vi "MainTester.vi"() -> ()   [LabVIEW 2015]
uses:
  <vilib>/Rock Robotics/WPI/SerialPort/WPI_SerialPortRef.ctl
  <vilib>/Rock Robotics/WPI/SerialPort/WPI_SerialPort.ctl
  Old code/packet types.ctl
panel:
  in  "B 2":dbl(slide) scale=0.0..255.0
  in  "G 2":dbl(slide) scale=0.0..255.0
  in  "R 2":dbl(slide) scale=0.0..255.0
  in  "B":dbl(slide) scale=0.0..255.0
  in  "G":dbl(slide) scale=0.0..255.0
  in  "R":dbl(slide) scale=0.0..255.0
  out "SerialPortRef 6":T1
  out "error out 8":errorcluster
  out "SerialPortRef":T1
  out "error out 7":errorcluster
  in  "Close File 2":bool
  in  "Close File":bool
  in  "Display string":string
  out "error out 6":errorcluster
  out "SerialPortRef 5":T1
  out "ADC voltages":dbl[](array[numeric])
  out "error out 4":errorcluster
  out "SerialPortRef 3":T1
  out "error out 3":errorcluster
  out "SerialPortRef 2":T1
  out "error out 2":errorcluster
  out "All Digital Input Vals":bool[](array[boolean])
  out "error out":errorcluster
  in  "stop":bool
  in  "error in (no error)":errorcluster
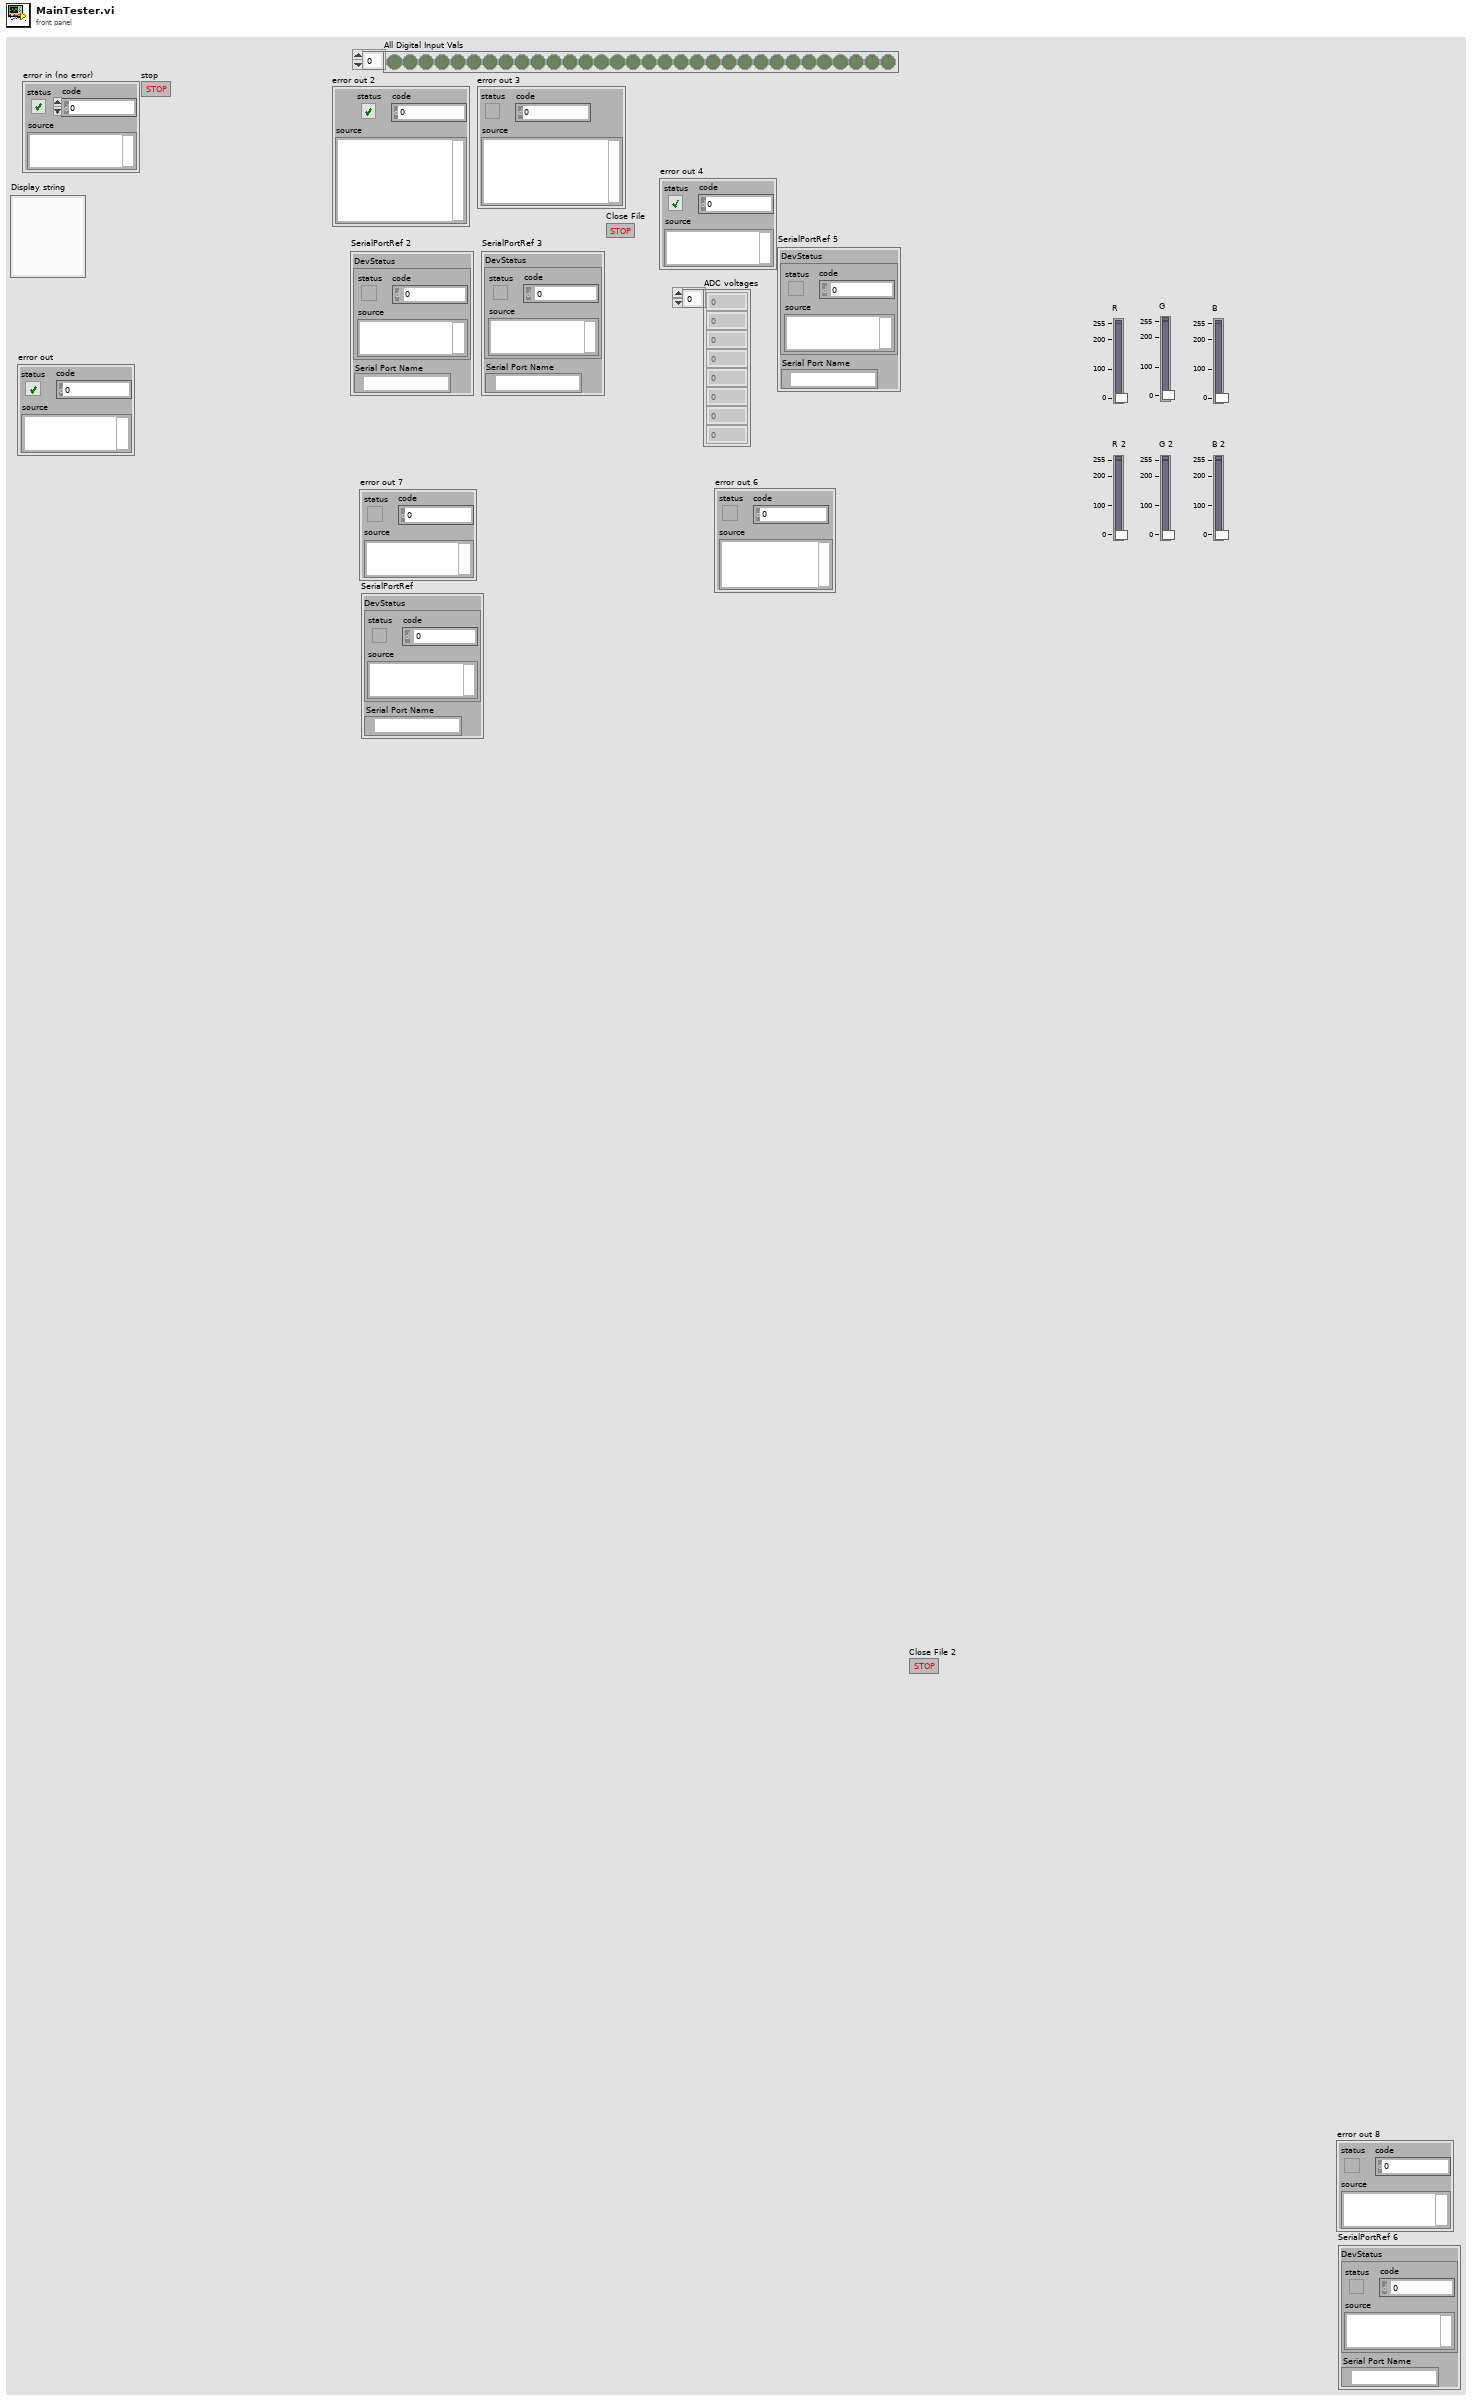
[diagram p1: front panel]
types:
  T1 = typedef "WPI_SerialPortRef.ctl" = cluster{"DevStatus":errorcluster, "Serial Port Name":refnum<visa-resource-name>}
  T2 = typedef "WPI_SerialPort.ctl" = enum16{"Onboard RS-232", "MXP TTL"}
  T3 = typedef "packet types.ctl" = enum16{"Log line", "Open File", "Close File", "Send Header", "Set Time", "Send to LCD"}
  T4 = enum16{"Set Custom RGB", "Set Mode", "Set intensity"}
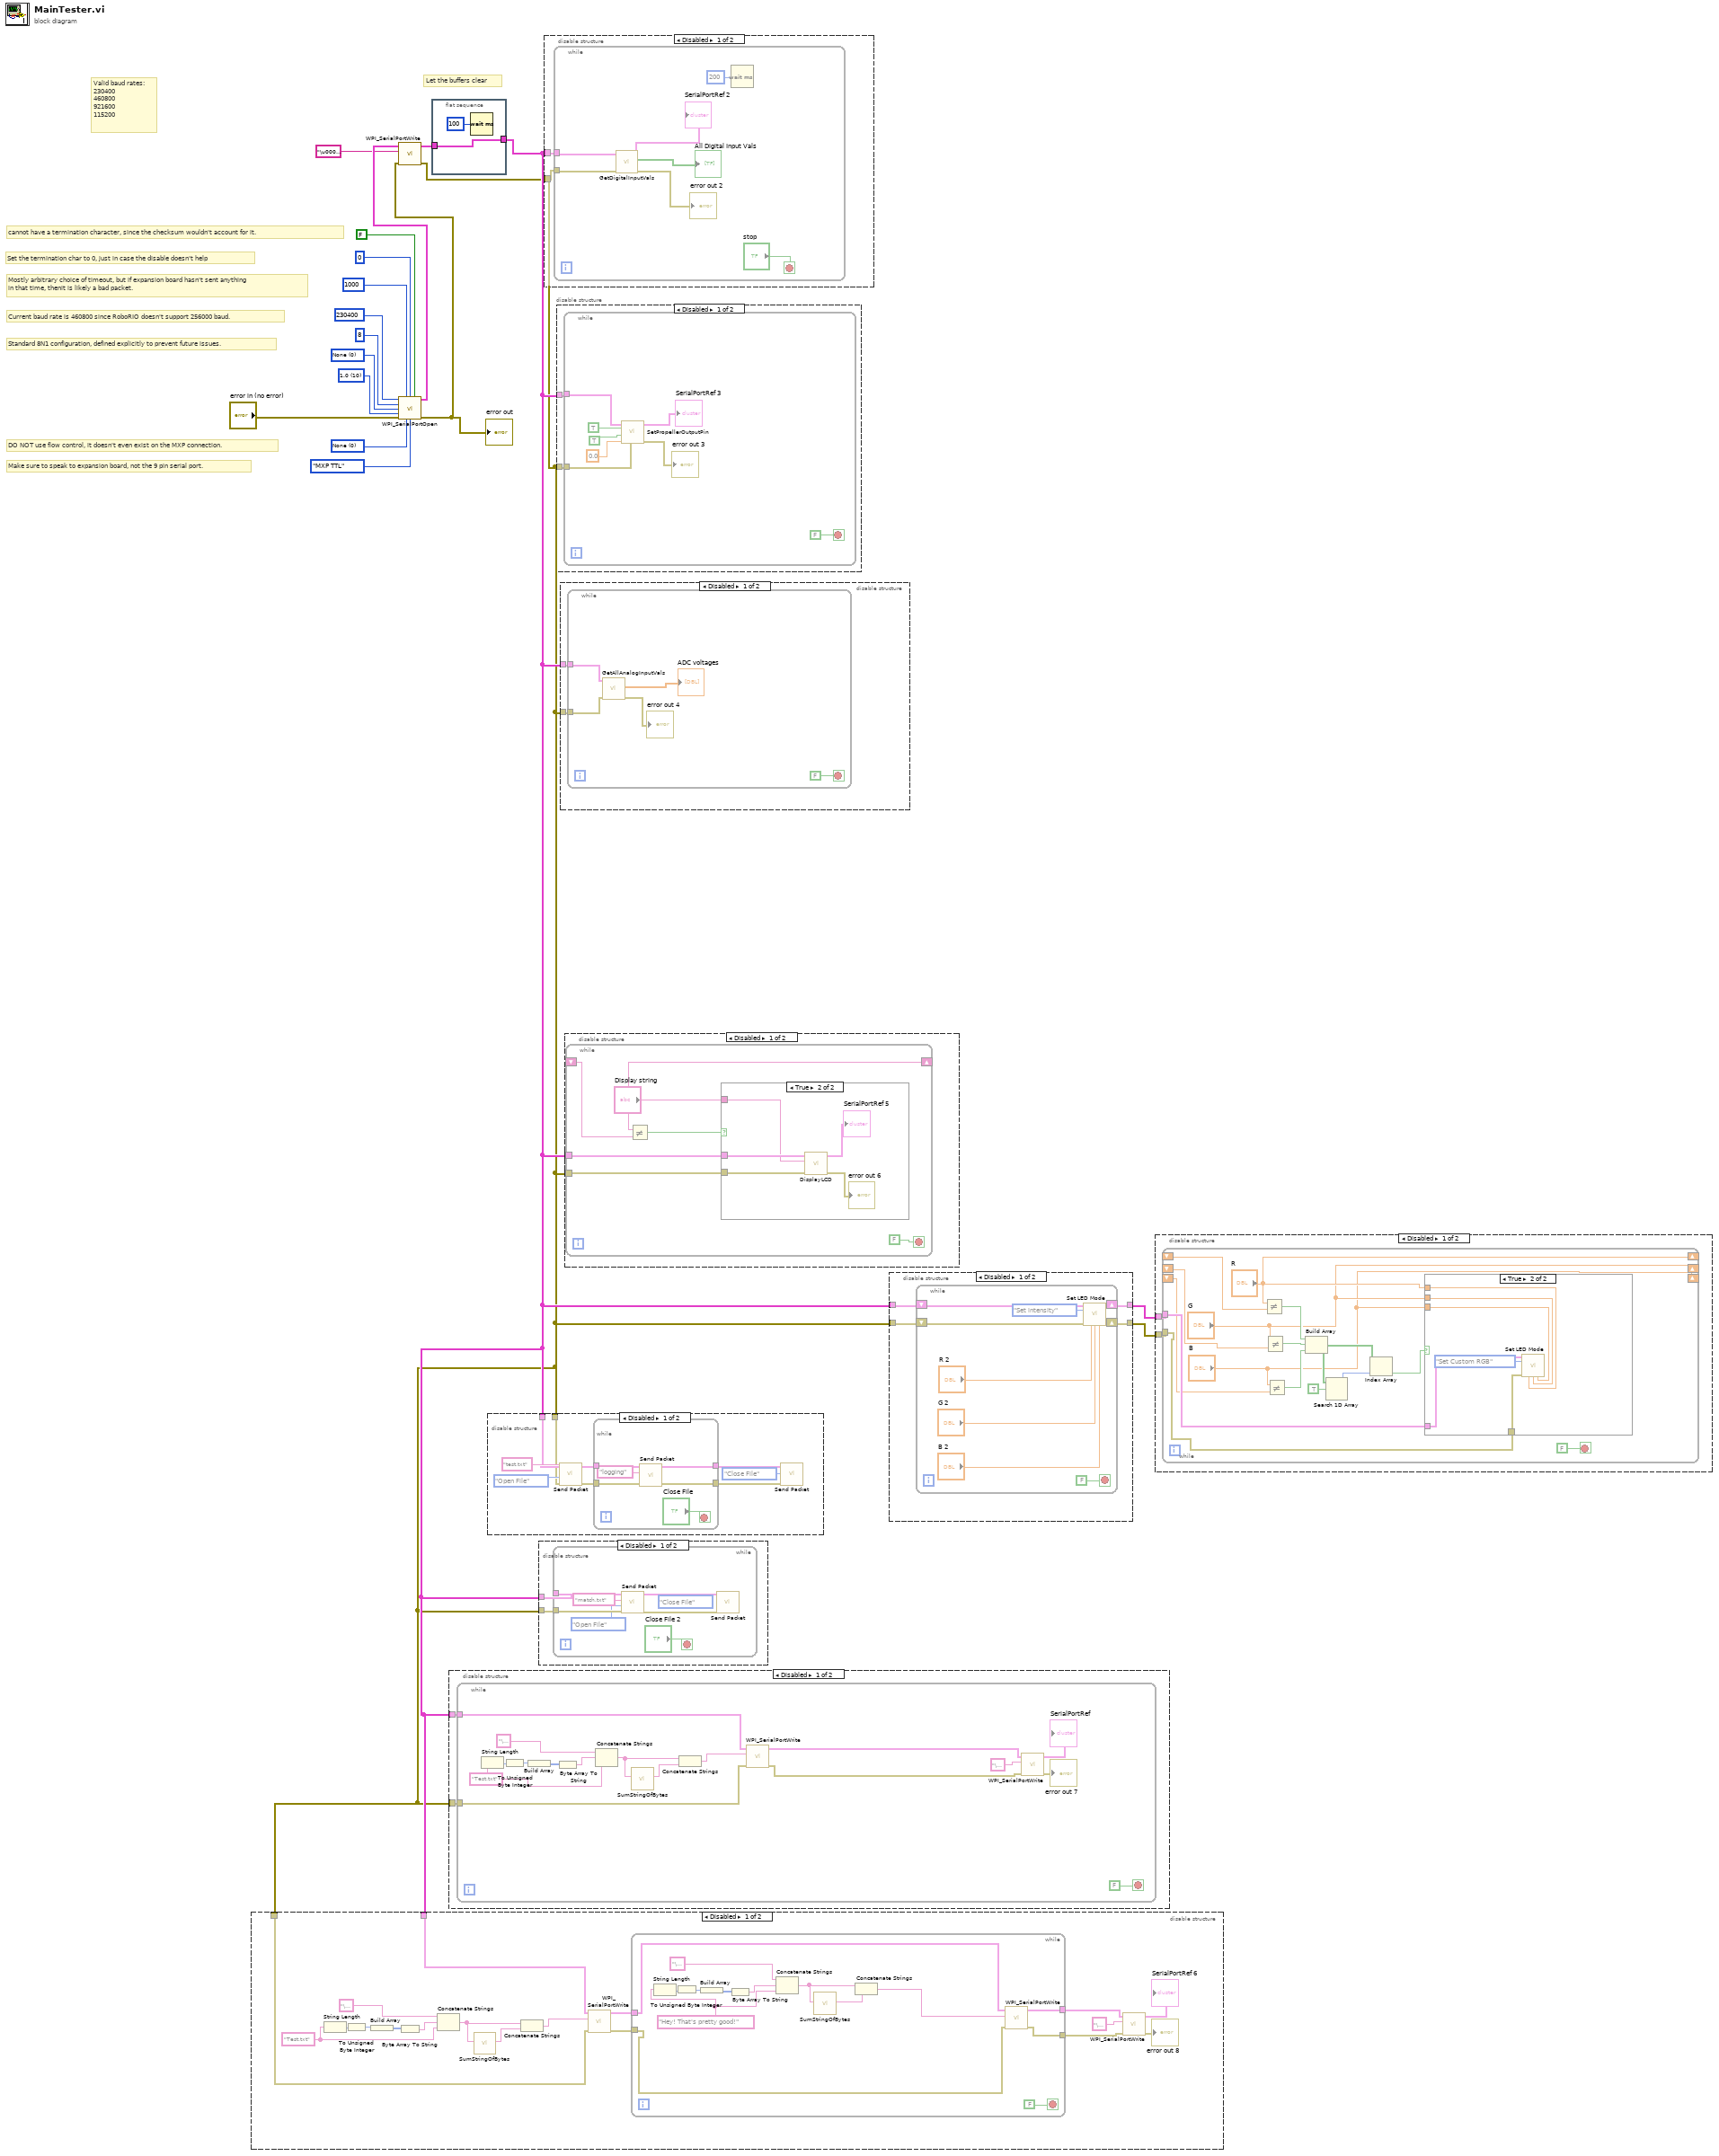
[diagram p0: block diagram]
diagram:
  w17 = u16 10 items=["1.0"=10, "1.5"=15, "2.0"=20] ("Stop Bits")
  w13 = u16 0 items=["None", "XON/XOFF", "RTS/CTS", "XON/XOFF & RTS/CTS", "DTR/DSR", "XON/XOFF & DTR/DSR"] ("Flow Control")
  w12 = u16 0 items=["None", "Odd", "Even", "Mark", "Space"] ("Parity")
  # "Let the buffers clear"
  # "Valid baud rates:\n230400\n460800\n921600\n115200"
  # "Make sure to speak to expansion board, not the 9 pin serial port."
  # "DO NOT use flow control, it doesn't even exist on the MXP connection."
  # "Standard 8N1 configuration, defined explicitly to prevent future issues."
  # "Current baud rate is 460800 since RoboRIO doesn't support 256000 baud."
  # "Mostly arbitrary choice of timeout, but if expansion board hasn't sent anything\nin that time, thenit is likely a bad packet."
  # "Set the termination char to 0, just in case the disable doesn't help"
  # "cannot have a termination character, since the checksum wouldn't account for it."
  n1 = call <vilib>:"WPI_SerialPortOpen.vi"("Baud Rate"=u32 230400, "Timeout Value (ms)"=u32 1000, "Termination Char (0xA = '\\n' = LF)"=u8 0 ("Termination Char (0xA = '\\n' = LF)"), "Enable Termination Char? (T)"=FALSE, "Data Bits"=u16 8, "Parity"=w12, "Stop Bits"=w17, "error in (no error)"="error in (no error)", "Flow Control"=w13, "Serial Port"=WPI_SerialPort."MXP TTL") -> ("SerialPortRef"=w8:T1, "error out"=w7:errorcluster)  [unwired: 4 in]
  "error out" <- w7
  n2 = call <vilib>:"WPI_SerialPortWrite.vi"("error in (no error)"=w7, "Buffer"="\u0004\u0004", "SerialPortRef"=w8) -> ("error out"=w1:errorcluster, "SerialPortRef"=w5:T1)  [unwired: 6 in, 1 out]
  n3 = disable-structure shown="Disabled" {
    disable-tunnel: w2 -> [w36 _]
    disable-tunnel: w1 -> [w35 _]
    frame Disabled {
      w19 = "Test.txt"
      n4 = String Length(string=w19) -> (length=w27:i32)
      n5 = To Unsigned Byte Integer(number=w27) -> (unsigned 8bit integer=w30:u8)
      n6 = Build Array(w30) -> (w29:u8[])
      n7 = Byte Array To String(unsigned byte array=w29) -> (string=w28:string)
      n8 = Concatenate Strings("\u0003", w28, w19) -> (w33:string)
      n9 = call "SumStringOfBytes.vi"("String Of Bytes"=w33) -> ("SumAsString"=w34:string)  [unwired: 10 in]
      n10 = Concatenate Strings(w33, w34) -> (w31:string)
      n11 = call <vilib>:"WPI_SerialPortWrite.vi"("error in (no error)"=w35, "Buffer"=w31, "SerialPortRef"=w36) -> ("error out"=w25:errorcluster, "SerialPortRef"=w26:T1)  [unwired: 6 in, 1 out]
      n12 = while {
        tunnel: w26 -> [w50]
        tunnel: w25 -> [w49]
        tunnel: [w39] -> w21
        tunnel: [w38] -> w20
        stop <- FALSE stop-if-true
        w43 = "Hey! That's pretty good!"
        n13 = String Length(string=w43) -> (length=w45:i32)
        n14 = To Unsigned Byte Integer(number=w45) -> (unsigned 8bit integer=w47:u8)
        n15 = Build Array(w47) -> (w46:u8[])
        n16 = Byte Array To String(unsigned byte array=w46) -> (string=w44:string)
        n17 = Concatenate Strings("\u0001", w44, w43) -> (w41:string)
        n18 = call "SumStringOfBytes.vi"("String Of Bytes"=w41) -> ("SumAsString"=w42:string)  [unwired: 10 in]
        n19 = Concatenate Strings(w41, w42) -> (w40:string)
        n20 = call <vilib>:"WPI_SerialPortWrite.vi"("error in (no error)"=w49, "Buffer"=w40, "SerialPortRef"=w50) -> ("error out"=w38:errorcluster, "SerialPortRef"=w39:T1)  [unwired: 6 in, 1 out]
      }
      n21 = call <vilib>:"WPI_SerialPortWrite.vi"("error in (no error)"=w20, "Buffer"="\u0004", "SerialPortRef"=w21) -> ("error out"=→"error out 8":errorcluster, "SerialPortRef"=→"SerialPortRef 6":T1)  [unwired: 6 in, 1 out]
    }
    frame Enabled {
    }
  }
  n22 = flat-sequence {
    tunnel: [w52] -> w2
    tunnel: w5 -> [w52]
    frame #0 {
      n23 = Wait (ms)(milliseconds to wait=u32 100) -> ()  [unwired: 1 out]
    }
  }
  n24 = disable-structure shown="Disabled" {
    disable-tunnel: w1 -> [w54 _]
    disable-tunnel: w2 -> [w53 _]
    frame Disabled {
      n25 = while {
        tunnel: w53 -> [w71]
        tunnel: w54 -> [w70]
        stop <- FALSE stop-if-true
        w61 = "Test.txt"
        n26 = String Length(string=w61) -> (length=w57:i32)
        n27 = To Unsigned Byte Integer(number=w57) -> (unsigned 8bit integer=w60:u8)
        n28 = Build Array(w60) -> (w59:u8[])
        n29 = Byte Array To String(unsigned byte array=w59) -> (string=w58:string)
        n30 = Concatenate Strings("\u0003", w58, w61) -> (w68:string)
        n31 = call "SumStringOfBytes.vi"("String Of Bytes"=w68) -> ("SumAsString"=w69:string)  [unwired: 10 in]
        n32 = Concatenate Strings(w68, w69) -> (w66:string)
        n33 = call <vilib>:"WPI_SerialPortWrite.vi"("error in (no error)"=w70, "Buffer"=w66, "SerialPortRef"=w71) -> ("error out"=w55:errorcluster, "SerialPortRef"=w56:T1)  [unwired: 6 in, 1 out]
        n34 = call <vilib>:"WPI_SerialPortWrite.vi"("error in (no error)"=w55, "Buffer"="\u0004", "SerialPortRef"=w56) -> ("error out"=→"error out 7":errorcluster, "SerialPortRef"=→"SerialPortRef":T1)  [unwired: 6 in, 1 out]
      }
    }
    frame Enabled {
    }
  }
  n35 = disable-structure shown="Disabled" {
    disable-tunnel: w2 -> [w73 _]
    disable-tunnel: w1 -> [w72 _]
    frame Disabled {
      n36 = call "Send Packet.vi"("error in (no error) 2"=w72, 7:packet_types."Open File", "Log string 2"="test.txt" ("Log string"), "SerialPortRef 2"=w73) -> ("error out 2"=w77:errorcluster, "SerialPortRef out 2"=w78:T1)  [unwired: 4 in]
      n37 = while {
        tunnel: w78 -> [w86]
        tunnel: w77 -> [w85]
        tunnel: [w82] -> w76
        tunnel: [w81] -> w75
        stop <- "Close File" stop-if-true
        n38 = call "Send Packet.vi"("error in (no error) 2"=w85, "Log string 2"="logging" ("Log string"), "SerialPortRef 2"=w86) -> ("error out 2"=w81:errorcluster, "SerialPortRef out 2"=w82:T1)  [unwired: 5 in]
      }
      n39 = call "Send Packet.vi"("error in (no error) 2"=w75, 7:packet_types."Close File", "SerialPortRef 2"=w76) -> ()  [unwired: 5 in, 2 out]
    }
    frame Enabled {
    }
  }
  n40 = disable-structure shown="Disabled" {
    disable-tunnel: w2 -> [w88 _]
    disable-tunnel: w1 -> [w87 _]
    frame Disabled {
      n41 = while {
        tunnel: w88 -> [w95]
        tunnel: w87 -> [w94]
        stop <- "Close File 2" stop-if-true
        (unwired) packet_types."Close File"
        n42 = call "Send Packet.vi"("error in (no error) 2"=w94, 7:packet_types."Open File", "Log string 2"="match.txt" ("Log string"), "SerialPortRef 2"=w95) -> ("error out 2"=w89:errorcluster, "SerialPortRef out 2"=w90:T1)  [unwired: 4 in]
        n43 = call "Send Packet.vi"("error in (no error) 2"=w89, "SerialPortRef 2"=w90) -> ()  [unwired: 6 in, 2 out]
      }
    }
    frame Enabled {
    }
  }
  n44 = disable-structure shown="Disabled" {
    disable-tunnel: w1 -> [w97 _]
    disable-tunnel: w2 -> [w96 _]
    frame Disabled {
      n45 = while {
        tunnel: w97 -> [w102]
        tunnel: w96 -> [w103]
        stop <- "stop" stop-if-true
        n46 = call "GetDigitalInputVals.vi"("error in (no error)"=w102, "SerialPortRef"=w103) -> ("error out"=→"error out 2":errorcluster, "All Digital Input Vals"=→"All Digital Input Vals":bool[], "SerialPortRef 2"=→"SerialPortRef 2":T1)  [unwired: 7 in]
        n47 = Wait (ms)(milliseconds to wait=u32 200) -> ()  [unwired: 1 out]
      }
    }
    frame Enabled {
    }
  }
  n48 = disable-structure shown="Disabled" {
    disable-tunnel: w1 -> [w106 _]
    disable-tunnel: w2 -> [w105 _]
    frame Disabled {
      n49 = while {
        tunnel: w106 -> [w111]
        tunnel: w105 -> [w108]
        stop <- FALSE stop-if-true
        n50 = call "SetPropellerOutputPin.vi"("error in (no error)"=w111, "Pin Number"=0.0, "Value"=TRUE, "Dir"=TRUE, "SerialPortRef"=w108) -> ("error out"=→"error out 3":errorcluster, "SerialPortRef 2"=→"SerialPortRef 3":T1)  [unwired: 5 in]
      }
    }
    frame Enabled {
    }
  }
  n51 = disable-structure shown="Disabled" {
    disable-tunnel: w2 -> [w116 _]
    disable-tunnel: w1 -> [w115 _]
    frame Disabled {
      n52 = while {
        tunnel: w116 -> [w121]
        tunnel: w115 -> [w120]
        stop <- FALSE stop-if-true
        n53 = call "GetAllAnalogInputVals.vi"("error in (no error)"=w120, "SerialPortRef"=w121) -> ("error out"=→"error out 4":errorcluster, "ADC voltages"=→"ADC voltages":dbl[])  [unwired: 6 in, 2 out]
      }
    }
    frame Enabled {
    }
  }
  n54 = disable-structure shown="Disabled" {
    disable-tunnel: w2 -> [w123 _]
    disable-tunnel: w1 -> [w122 _]
    frame Disabled {
      n55 = while {
        tunnel: w123 -> [w127]
        tunnel: w122 -> [w129]
        shift-right: ["Display string"] -> _
        shift-left: _ -> [w125]
        stop <- FALSE stop-if-true
        n56 = Not Equal?(x="Display string", y=w125) -> (x != y?=w124:bool)
        n57 = case shown="True" w124 {
          tunnel: w127 -> [_ w134]
          tunnel: w129 -> [_ w133]
          tunnel: "Display string" -> [_ w130]
          frame False {
          }
          frame True {
            n58 = call "DisplayLCD.vi"("error in (no error)"=w133, "Display string"=w130, "SerialPortRef"=w134) -> ("error out"=→"error out 6":errorcluster, "SerialPortRef 2"=→"SerialPortRef 5":T1)  [unwired: 7 in]
          }
        }
      }
    }
    frame Enabled {
    }
  }
  n59 = disable-structure shown="Disabled" {
    disable-tunnel: w1 -> [w138 _]
    disable-tunnel: w2 -> [w137 _]
    disable-tunnel: [w136 _] -> w4
    disable-tunnel: [w135 _] -> w3
    frame Disabled {
      n60 = while {
        shift-right: [w144] -> w135
        shift-left: w138 -> [w147]
        shift-right: [w145] -> w136
        shift-left: w137 -> [w146]
        stop <- FALSE stop-if-true
        n61 = call "Set LED Mode.vi"("SerialPortRef 3"=w146, 5:T4."Set intensity" ("Enum"), "error in (no error)"=w147, "Red"="R 2", "Green"="G 2", "Blue"="B 2") -> ("SerialPortRef"=w145:T1, "error out"=w144:errorcluster)  [unwired: 8 in]
      }
    }
    frame Enabled {
    }
  }
  n62 = disable-structure shown="Disabled" {
    disable-tunnel: w4 -> [w149 _]
    disable-tunnel: w3 -> [w148 _]
    frame Disabled {
      n63 = while {
        tunnel: w149 -> [w163]
        tunnel: w148 -> [w164]
        shift-right: ["R"] -> _
        shift-left: _ -> [w162]
        shift-right: ["G"] -> _
        shift-left: _ -> [w161]
        shift-right: ["B"] -> _
        shift-left: _ -> [w160]
        stop <- FALSE stop-if-true
        n64 = Not Equal?(x="R", y=w162) -> (x != y?=w157:bool)
        n65 = Not Equal?(x="G", y=w161) -> (x != y?=w159:bool)
        n66 = Not Equal?(x="B", y=w160) -> (x != y?=w158:bool)
        n67 = Build Array(w157, w159, w158) -> (w154:bool[])
        n68 = Search 1D Array(1D array=w154, element=TRUE) -> (index of element=w155:i32)  [unwired: 1 in]
        n69 = Index Array(array=w154, index=w155) -> (element=w153:bool)
        n70 = case shown="True" w153 {
          tunnel: w164 -> [_ w170]
          tunnel: w163 -> [_ w171]
          tunnel: "R" -> [_ w166]
          tunnel: "G" -> [_ w167]
          tunnel: "B" -> [_ w168]
          frame False {
          }
          frame True {
            n71 = call "Set LED Mode.vi"("SerialPortRef 3"=w171, 5:enum16{"Set Custom RGB", "Set Mode"}."Set Custom RGB" ("Enum"), "error in (no error)"=w170, "Red"=w166, "Green"=w167, "Blue"=w168) -> ()  [unwired: 8 in, 2 out]
          }
        }
      }
    }
    frame Enabled {
    }
  }
